vi "DB Open.vi"(8 "error in (no error)":errorcluster, 9 "Password":string, 10 "UserID":string, 11 "dbpath":string) -> (0 "error out":errorcluster, 3 "Db Reference Out":refnum<k24>)   [LabVIEW 2020]
uses:
  D:/Labview/Auto Run Screen/Source Code/Database/Support/dbquery.dll
  Support/dbquery.dll
panel:
  out "opendb":string
  in  "ConnectionString":string
  out "Automation Refnum out":refnum<k7>
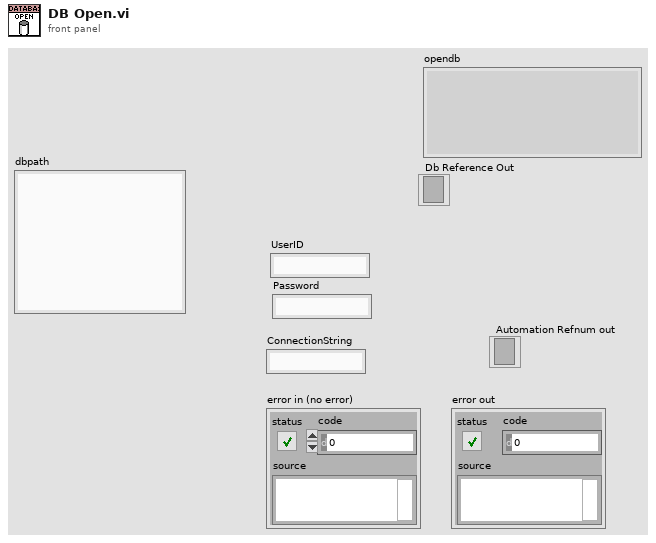
[diagram p1: front panel]
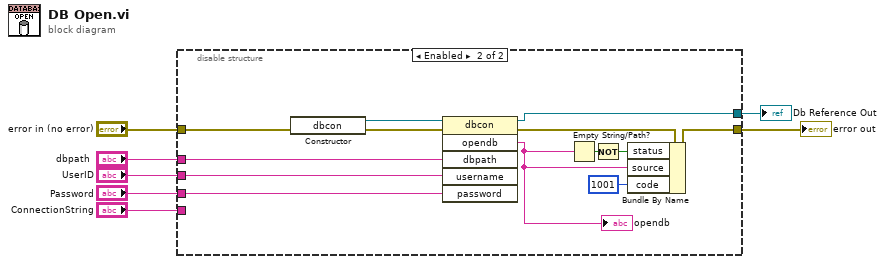
[diagram p0: block diagram]
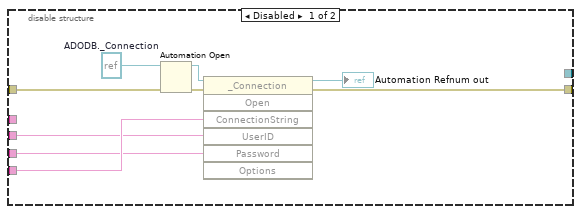
[diagram p2: hidden frame]
diagram:
  n1 = disable-structure shown="Enabled" {
    disable-tunnel: "error in (no error)" -> [w16 w26]
    disable-tunnel: [w14 w23] -> w6
    disable-tunnel: "ConnectionString" -> [w12 _]
    disable-tunnel: "UserID" -> [w9 w28]
    disable-tunnel: "Password" -> [w8 w27]
    disable-tunnel: "dbpath" -> [_ w17]
    disable-tunnel: [_ w18] -> w1
    frame Disabled {
      w10 = refnum<k7> refnum  # ADODB._Connection
      n2 = Automation Open(error in (no error)=w16, Automation Refnum=w10) -> (Automation Refnum=w11:refnum<k7>, error out=w15:errorcluster)  [unwired: 2 in]
      n3 = invoke class="_Connection" method="Open"(reference=w11, error in=w15, "ConnectionString"=w12, "UserID"=w9, "Password"=w8) -> (reference out=→"Automation Refnum out":refnum<k7>, error out=w14:errorcluster)  [unwired: 2 in, 5 out]
    }
    frame Enabled {
      n4 = constructor class="dbcon"(error in=w26) -> (reference out=w29:refnum<k24>, error out=w25:errorcluster)  [unwired: 2 in, 1 out]
      n5 = invoke class="dbcon" method="opendb"(reference=w29, error in=w25, "dbpath"=w17, "username"=w28, "password"=w27) -> (reference out=w18:refnum<k24>, error out=w24:errorcluster, "opendb"=w20:string)  [unwired: 1 in, 3 out]
      "opendb" <- w20
      n6 = Empty String/Path?(string/path=w20) -> (empty?=w22:bool)
      n7 = Not(x=w22) -> (.not. x?=w21:bool)
      n8 = Bundle By Name(cluster=w24, "status"=w21, "source"=w20, "code"=1001) -> (w23:errorcluster)
    }
  }
  "error out" <- w6
  "Db Reference Out" <- w1
